vi "SVA 4MV5 PF CCSA RPJ SLJC.vi"() -> ()   [LabVIEW 2021]
uses:
  Control-Case.ctl
  <vilib>/vision/Image Controls.llb/IMAQ Image.ctl
  <vilib>/vision/NI_Vision_Development_Module.lvlib
panel:
  out "Aprobación de Lata":bool
  out "Distance 2":dbl[](graph) caption="Distancia entre perfil ideal y perfil real"
  out "Distance":dbl[](graph) caption="Distancia entre perfil ideal y perfil real"
  out "new picture 2":picture
  out "new picture":picture
  out "Datos finales":T1(array[cluster])
  in  "Crear patrón":bool
  in  "Concluir":bool
  in  "Lateral":bool
  in  "Superior":bool
  out "Fecha final":timestamp
  out "Rechazadas":dbl
  out "Aprobadas":dbl
  in  "Valor de aprobación Superiror":dbl=4.0 min=0.0 format="%.2f"
  out "Fecha inicio":timestamp
  out "Muestras":i32
  in  "Valor de aprobación Frontal":dbl=4.0 min=0.0 format="%.2f"
  # "Descripción:\nEste instrumento virtual permite detectar irregularidades en la geometría de latas de refresco usando el análisis de contornos:\n-Primeramente debe obtenerse un patrón para el perfil lateral e caso de no tenerlo, pues este se usará para detectar las irregularidades de capturas posteriores.\n-Como siguiente paso se toma una captura del perfil lateral y esta se desplegará en la imagen izquierda.\n-Como siguiente paso se toma una captura del perfil superior y esta se desplegará en la imagen derecha."
  # "Sistema de detección de defectos en latas \nbasado en el análisis de contornos\nProyecto de fin de semestre \nSistemas de visión artificial\nProfesor Erick Huitrón Ramírez"
  # "CUEVAS CERÓN SERGIO ALBERTO\nREYES PÉREZ JAVIER\nSALCEDO LICEA JUAN CARLOS"
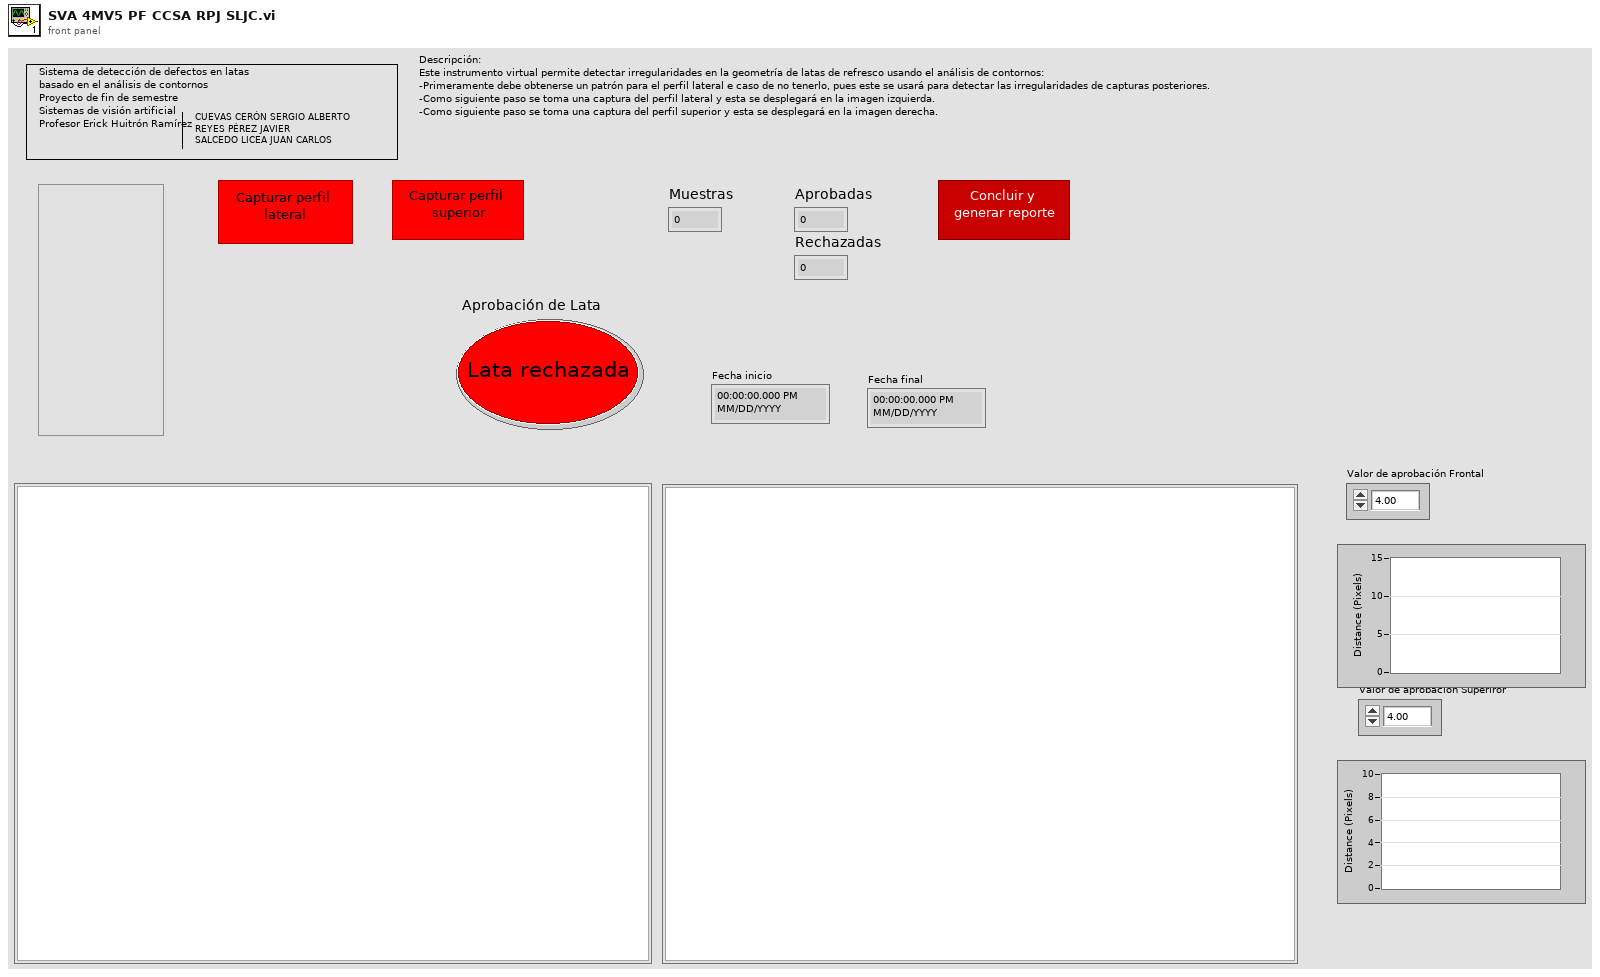
[diagram p1: front panel]
types:
  T1 = cluster{"Class":string, string, string, string}[]
  T2 = typedef "IMAQ Image.ctl" = refnum<image>
  T3 = typedef "Control-Case.ctl" = enum16{"Espera", "Patrón", "Toma lateral", "Toma superior", "Concluir"}
  T4 = enum16{"Rect Left To Right", "Rect Right To Left", "Rect Top To Bottom", "Rect Bottom To Top", "Annulus Inner To Outer", "Annulus Outer To Inner", "Annulus Start Angle To End Angle", "Annulus End Angle To Start Angle"}
  T5 = enum16{"Closest To Search Start", "Maximum Length", "Strongest Mean Gradient Change"}
  T6 = cluster{"Overlay?":bool, "Color":u32, "Width":u32, "Maintain Width?":bool}
  T7 = typedef "IMAQ Rectangle" = cluster{"Left":i32, "Top":i32, "Right":i32, "Bottom":i32, "Rotation":dbl}
  T8 = typedef "ROI Descriptor" = cluster{"Global Rectangle":i32[], "Contours":cluster{"ID":enum32{"External", "Internal"}, "Type":u32, "Coordinates":i32[]}[]}
  T9 = cluster{"Distance (Pixels)":dbl, "Distance (Real World)":dbl, "Angle (Absolute)":dbl, "Angle (Relative)":dbl}
  T10 = cluster{"Target Point":cluster{"X":dbl, "Y":dbl}, "Template Point":cluster{"X":dbl, "Y":dbl}, "Distance":dbl}[]
  T11 = cluster{"Center":cluster{"X":sgl, "Y":sgl}, "Radius":dbl, "Start Angle":dbl, "End Angle":dbl}
  T12 = cluster{"Class":string, "Distance (Pixels)":dbl, bool, dbl}
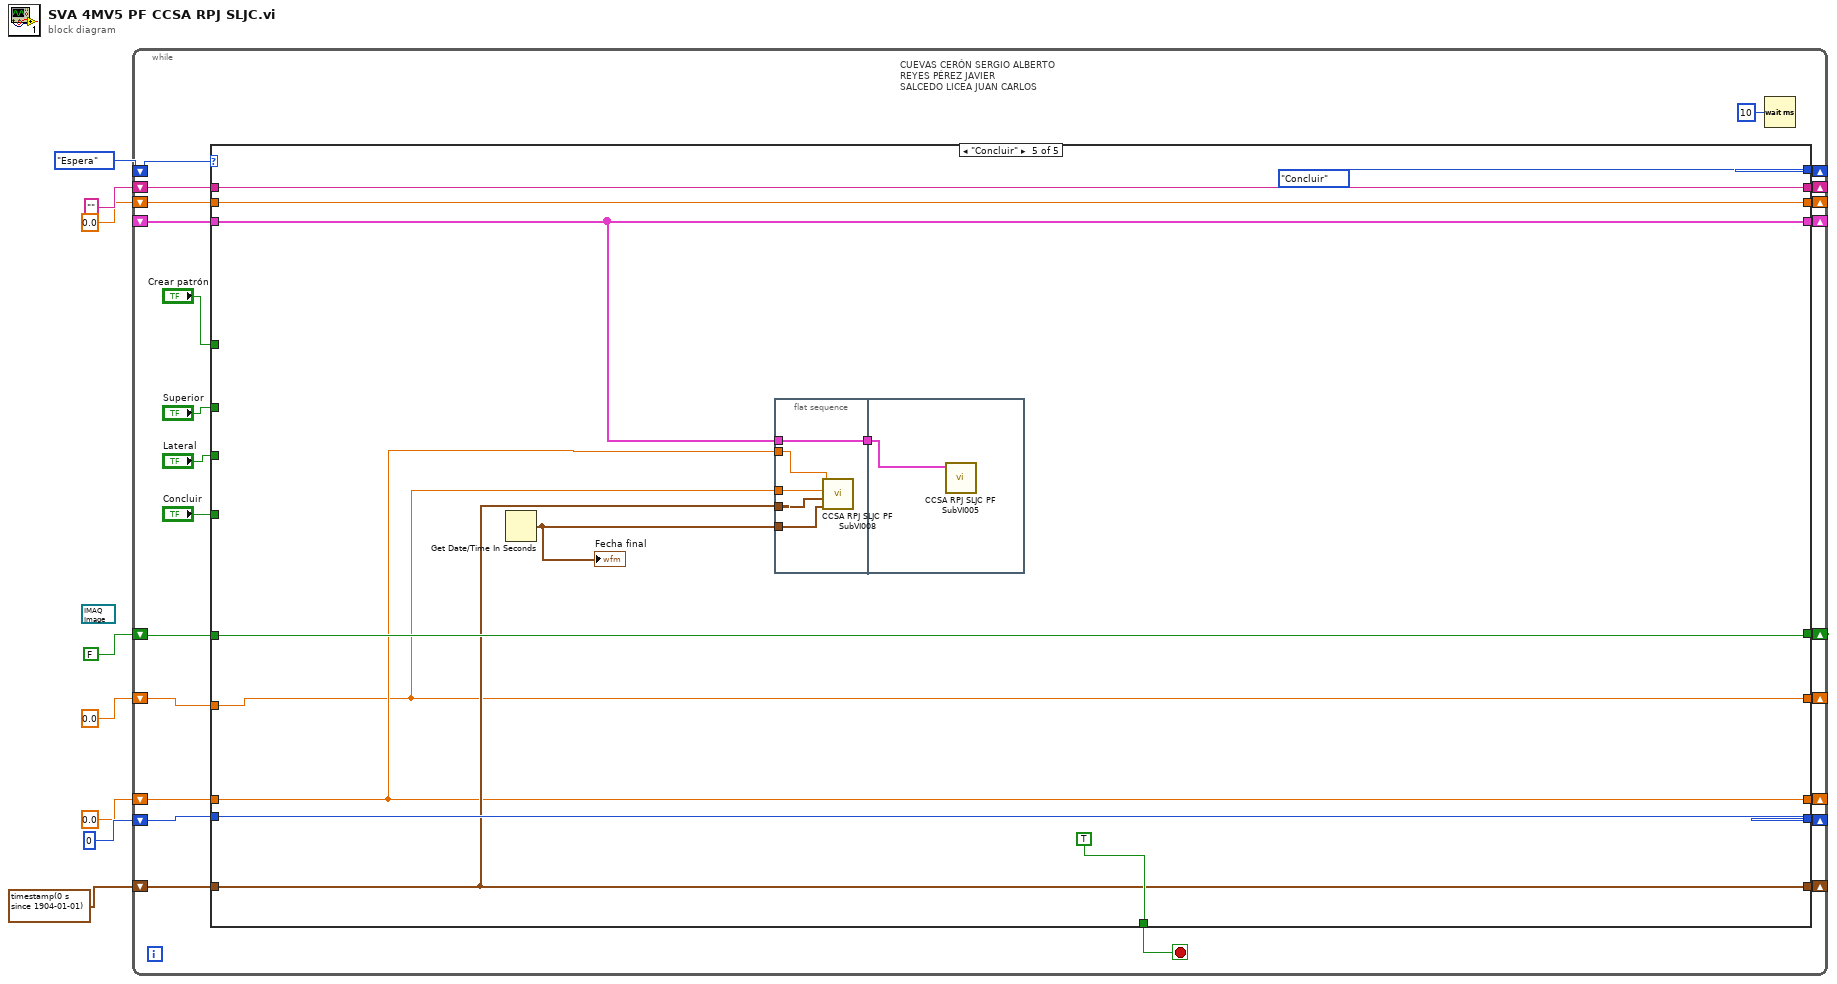
[diagram p0: block diagram]
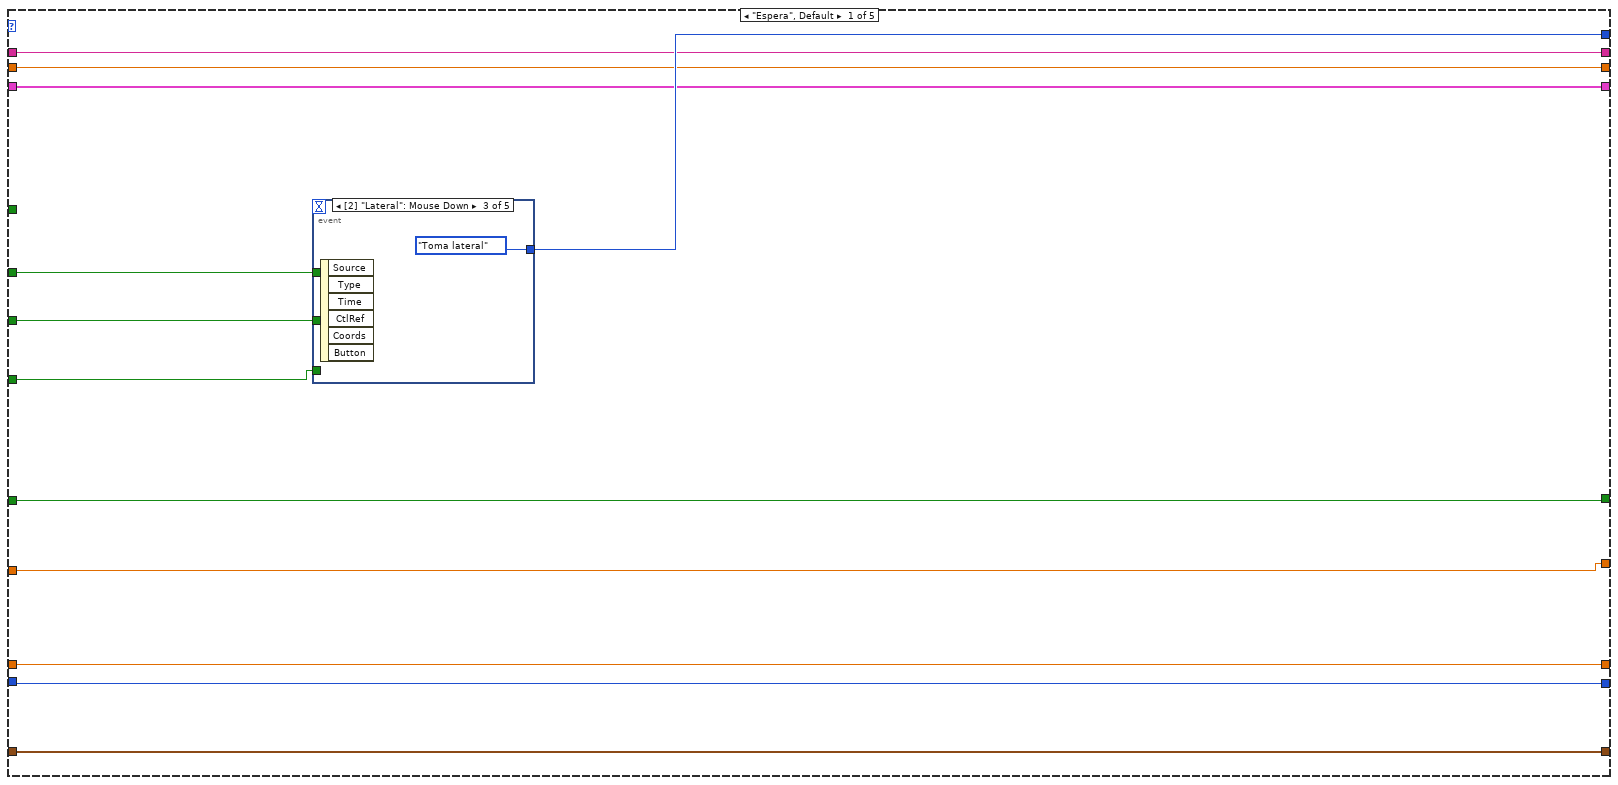
[diagram p2: hidden frame]
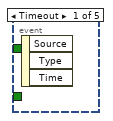
[diagram p3: hidden frame]
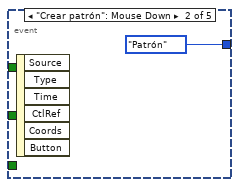
[diagram p4: hidden frame]
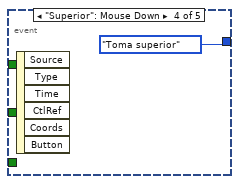
[diagram p5: hidden frame]
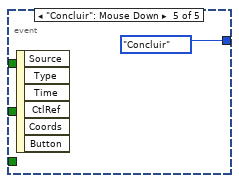
[diagram p6: hidden frame]
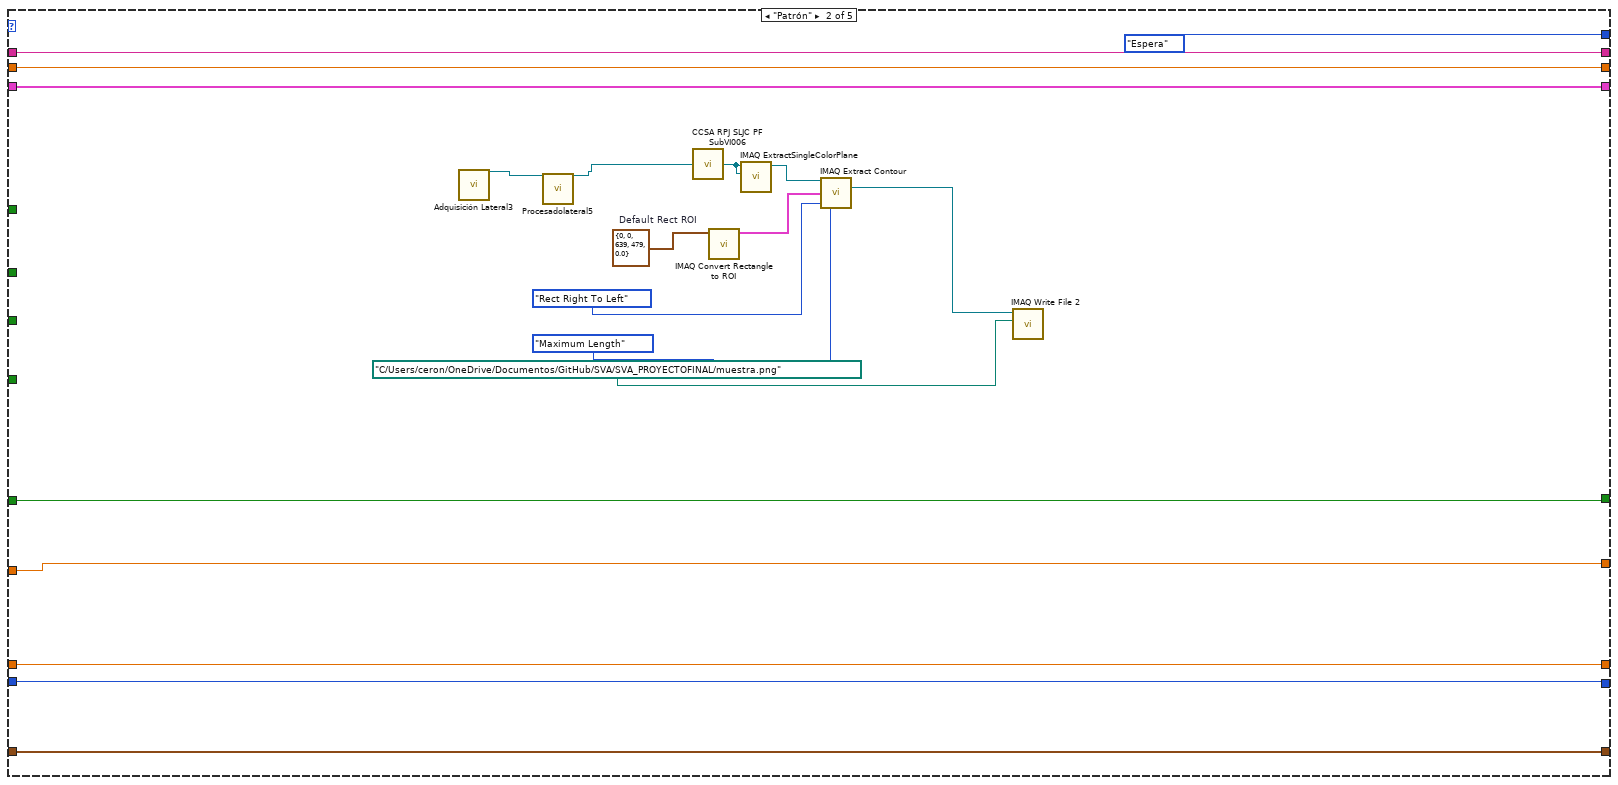
[diagram p7: hidden frame]
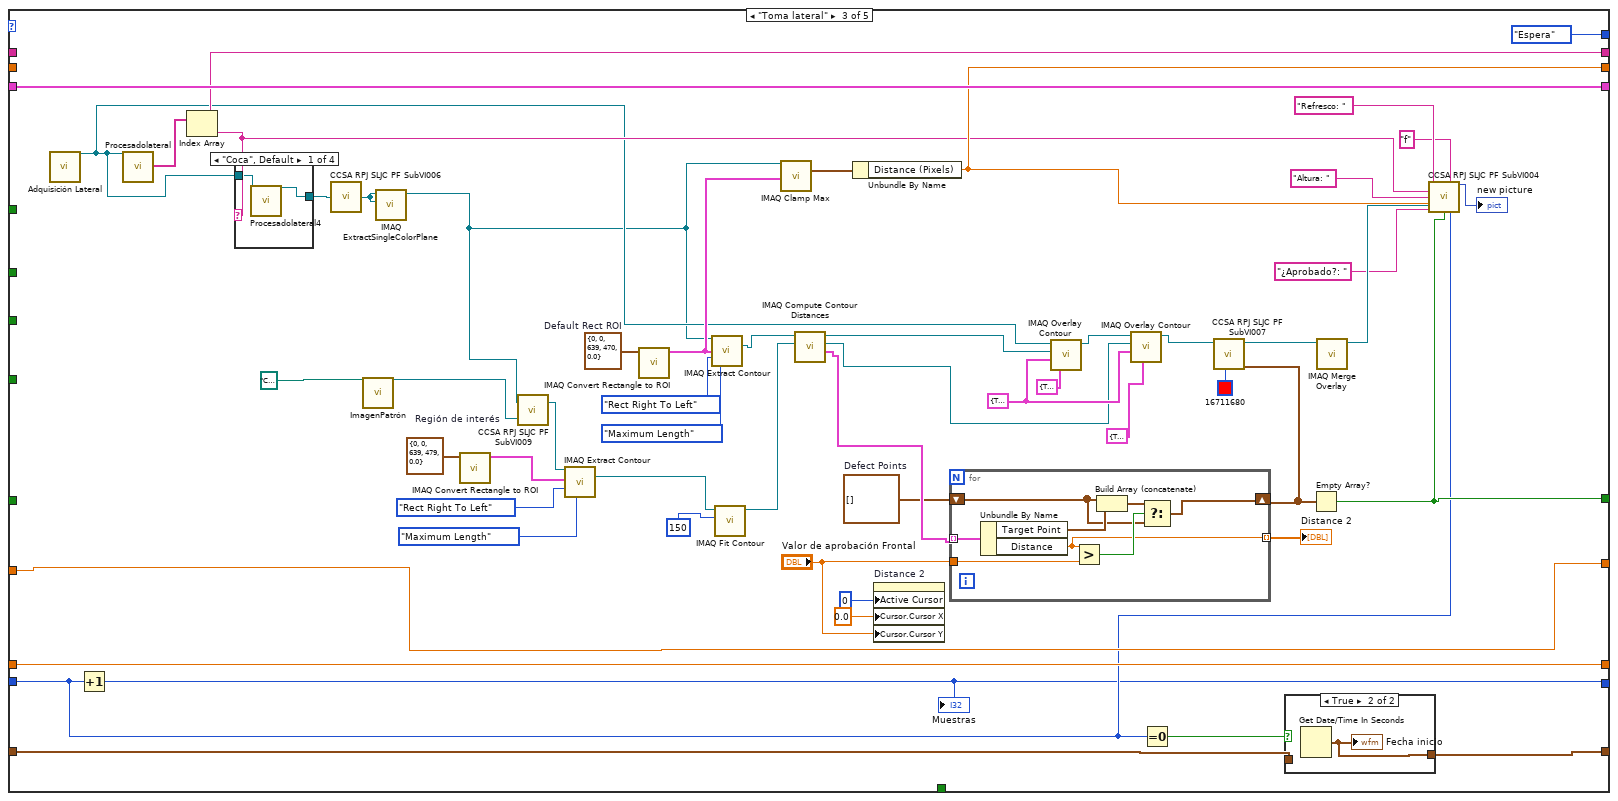
[diagram p8: hidden frame]
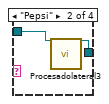
[diagram p10: hidden frame]
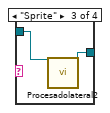
[diagram p11: hidden frame]
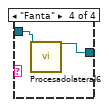
[diagram p12: hidden frame]
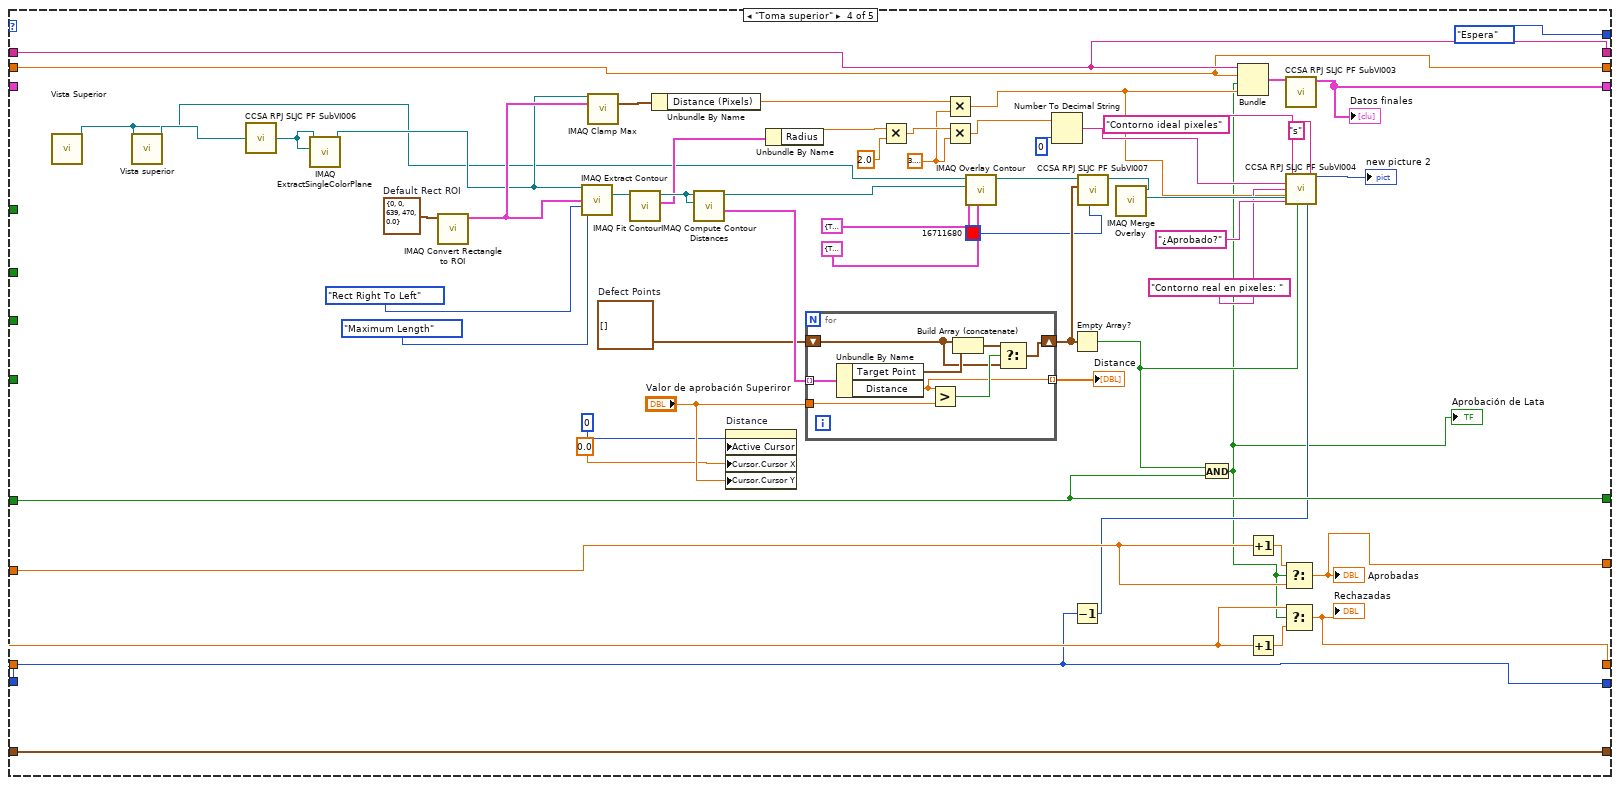
[diagram p13: hidden frame]
diagram:
  (unwired) T2 refnum ("Image Out (duplicate)")
  n1 = while {
    shift-right: [w32] -> _
    shift-left: Control-Case."Espera" -> [w31]
    shift-right: [w26] -> _
    shift-left: 0 ("x") -> [w25]
    shift-right: [w24] -> _
    shift-left: FALSE ("empty?") -> [w23]
    shift-right: [w22] -> _
    shift-left: 0.0 -> [w20]
    shift-right: [w21] -> _
    shift-left: 0.0 -> [w19]
    shift-right: [w17] -> _
    shift-left: 0.0 ("Distance (Pixels)") -> [w15]
    shift-right: [w18] -> _
    shift-left: "" ("Class") -> [w16]
    shift-right: [w14] -> _
    shift-left: _ -> [w13]
    shift-right: [w12] -> _
    shift-left: timestamp(0 s since 1904-01-01) ("seconds since 1Jan1904") -> [w11]
    stop <- w30 stop-if-true
    # "CUEVAS CERÓN SERGIO ALBERTO\nREYES PÉREZ JAVIER\nSALCEDO LICEA JUAN CARLOS"
    n2 = case shown="\"Concluir\"" w31 {
      tunnel: [w44 Control-Case."Espera" Control-Case."Espera" Control-Case."Espera" Control-Case."Concluir"] -> w32
      tunnel: [_ _ _ _ TRUE] -> w30
      tunnel: "Concluir" -> [w43 _ _ _ _]
      tunnel: "Lateral" -> [w42 _ _ _ _]
      tunnel: "Superior" -> [w41 _ _ _ _]
      tunnel: w25 -> [w37 w55 w75 w142 w214]
      tunnel: [w37 w55 w71 w142 w214] -> w26
      tunnel: [w40 w58 w82 w173 w213] -> w24
      tunnel: w23 -> [w40 w58 _ w173 w213]
      tunnel: [w39 w57 w93 w168 w206] -> w22
      tunnel: [w38 w56 w92 w167 w207] -> w21
      tunnel: w20 -> [w39 w57 w93 w175 w206]
      tunnel: w19 -> [w38 w56 w92 w174 w207]
      tunnel: [w36 w54 w84 w172 w212] -> w18
      tunnel: [w35 w53 w85 w171 w211] -> w17
      tunnel: w16 -> [w36 w54 _ w172 w212]
      tunnel: w15 -> [w35 w53 _ w171 w211]
      tunnel: [w34 w52 w86 w170 w209] -> w14
      tunnel: w13 -> [w34 w52 w86 _ w209]
      tunnel: [w33 w51 w91 w169 w208] -> w12
      tunnel: w11 -> [w33 w51 w90 w169 w208]
      tunnel: "Crear patrón" -> [_ _ _ _ _]
      frame "Espera", Default {
        n3 = event shown="[2] \"Lateral\": Mouse Down" {
          selector: _ -> [_ _ _ _ _]
          dyn-events: _ -> [_ _ _ _ _]
          timeout: _ -> [_ _ _ _ _]
          tunnel: w41 -> [_ _ _ _ _]
          tunnel: w42 -> [_ _ _ _ _]
          tunnel: w43 -> [_ _ _ _ _]
          tunnel: [_ Control-Case."Patrón" Control-Case."Toma lateral" Control-Case."Toma superior" Control-Case."Concluir"] -> w44
          event Timeout {
            n4 = event-data() -> ()  [unwired: 1 in, 3 out]
          }
          event "Crear patrón": Mouse Down {
            n5 = event-data() -> ()  [unwired: 1 in, 6 out]
          }
          event "Lateral": Mouse Down {
            n6 = event-data() -> ()  [unwired: 1 in, 6 out]
          }
          event "Superior": Mouse Down {
            n7 = event-data() -> ()  [unwired: 1 in, 6 out]
          }
          event "Concluir": Mouse Down {
            n8 = event-data() -> ()  [unwired: 1 in, 6 out]
          }
        }
      }
      frame "Patrón" {
        w64 = T7 {"Left"=0, "Top"=0, "Right"=639, "Bottom"=479, "Rotation"=0.0}  # Default Rect ROI
        n9 = call "Adquisición Lateral3"() -> ("Image Out"=w50:T2)  [unwired: 26 in, 1 out]
        n10 = call "Procesadolateral5"("Image In"=w50) -> ("Image Out"=w49:T2)  [unwired: 25 in, 1 out]
        n11 = call "CCSA RPJ SLJC PF SubVI006.vi"("Refnum in"=w49) -> ("Refnum out"=w60:T2)
        n12 = call "IMAQ Convert Rectangle to ROI"("Rectangle"=w64) -> ("ROI Descriptor"=w63:T8)  [unwired: 8 in, 1 out]
        n13 = call "IMAQ ExtractSingleColorPlane"("Image Dst"=w60, "Image Src"=w60) -> ("Image Dst Out"=w67:T2)  [unwired: 8 in, 1 out]
        n14 = call "IMAQ Extract Contour"("Source Image"=w67, "ROI Descriptor"=w63, "Search Direction"=T4."Rect Right To Left", "Contour Selection"=T5."Maximum Length") -> ("Contour Image Out"=w62:T2)  [unwired: 4 in, 7 out]
        n15 = call-poly "IMAQ Write File 2"("File Path"=path "C:/Users/ceron/OneDrive/Documentos/GitHub/SVA/SVA_PROYECTOFINAL/muestra.png" ("Imagen \nPatrón 2"), "Image"=w62) -> ()  [unwired: 8 in, 2 out]
      }
      frame "Toma lateral" {
        w95 = T7 {"Left"=0, "Top"=0, "Right"=639, "Bottom"=479, "Rotation"=0.0}  # Región de interés
        w96 = T7 {"Left"=0, "Top"=0, "Right"=639, "Bottom"=470, "Rotation"=0.0}  # Default Rect ROI
        w108 = cluster{"X":dbl, "Y":dbl}[] []  # Defect Points
        w104 = T6 {"Overlay?"=TRUE, "Color"=6618880, "Width"=3, "Maintain Width?"=TRUE} ("Contour Points Settings")
        n16 = call "Adquisición Lateral"() -> ("Image Out"=w70:T2)  [unwired: 26 in, 1 out]
        n17 = Increment(x=w75) -> (x+1=w71:i32)
        "Muestras" <- w71
        n18 = call "Procesadolateral"("Image In"=w70) -> ("Classes (TipoRefresco)"=w120:string[])  [unwired: 23 in, 3 out]
        n19 = Index Array(array=w120) -> (element=w84:string)  [unwired: 1 in]
        n20 = case shown="\"Coca\", Default" w84 {
          tunnel: w70 -> [w133 w136 w137 w139]
          tunnel: [w134 w135 w138 w140] -> w121
          frame "Coca", Default {
            n21 = call "Procesadolateral4"("Image In"=w133) -> ("Image Out"=w134:T2)  [unwired: 25 in, 1 out]
          }
          frame "Pepsi" {
            n22 = call "Procesadolateral3"("Image In"=w136) -> ("Image Out"=w135:T2)  [unwired: 25 in, 1 out]
          }
          frame "Sprite" {
            n23 = call "Procesadolateral2"("Image In"=w137) -> ("Image Out"=w138:T2)  [unwired: 25 in, 1 out]
          }
          frame "Fanta" {
            n24 = call "Procesadolateral6"("Image In"=w139) -> ("Image Out"=w140:T2)  [unwired: 25 in, 1 out]
          }
        }
        n25 = call "CCSA RPJ SLJC PF SubVI006.vi"("Refnum in"=w121) -> ("Refnum out"=w115:T2)
        n26 = call "ImagenPatrón"("Image Path"=path "C:/Users/ceron/OneDrive/Documentos/GitHub/SVA/SVA_PROYECTOFINAL/muestra.png" ("Imagen \nPatrón")) -> ("Image Out"=w73:T2)  [unwired: 25 in, 1 out]
        n27 = call "IMAQ ExtractSingleColorPlane"("Image Dst"=w115, "Image Src"=w115) -> ("Image Dst Out"=w69:T2)  [unwired: 8 in, 1 out]
        n28 = call "IMAQ Convert Rectangle to ROI"("Rectangle"=w95) -> ("ROI Descriptor"=w117:T8)  [unwired: 8 in, 1 out]
        n29 = call "CCSA RPJ SLJC PF SubVI009.vi"("Patrón original"=w73, "Toma original"=w69) -> ("Patrón corregido"=w72:T2)  [unwired: 1 out]
        n30 = call "IMAQ Extract Contour"("Source Image"=w72, "ROI Descriptor"=w117, "Search Direction"=T4."Rect Right To Left", "Contour Selection"=T5."Maximum Length") -> ("Contour Image Out"=w78:T2)  [unwired: 4 in, 7 out]
        n31 = call "IMAQ Convert Rectangle to ROI"("Rectangle"=w96) -> ("ROI Descriptor"=w118:T8)  [unwired: 8 in, 1 out]
        n32 = call "IMAQ Extract Contour"("Source Image"=w69, "ROI Descriptor"=w118, "Search Direction"=T4."Rect Right To Left", "Contour Selection"=T5."Maximum Length") -> ("Contour Image Out"=w110:T2)  [unwired: 4 in, 7 out]
        n33 = call-poly "IMAQ Fit Contour"("Control Points"=u32 150, "Contour Image"=w78) -> ("Contour Image Out"=w77:T2)  [unwired: 2 in, 7 out]
        n34 = call "IMAQ Clamp Max"("Source Image"=w69, "ROI Descriptor"=w118) -> ("Clamp Results"=w119:T9)  [unwired: 8 in, 5 out]
        n35 = call "IMAQ Compute Contour Distances"("Template Contour Image"=w77, "Target Contour Image"=w110) -> ("Distances"=w112:T10, "Template Contour Image Out (dup)"=w76:T2, "Target Contour Image Out (dup)"=w114:T2)  [unwired: 3 in, 4 out]
        n36 = Unbundle By Name(w119) -> ("Distance (Pixels)"=w85:dbl)
        n37 = property on="Distance 2" class="WFGraph (strict)"("Active Cursor"=u32 0, "Cursor.Cursor X"=0.0 ("Cursor.Cursor Position:Cursor X"), "Cursor.Cursor Y"="Valor de aprobación Frontal") -> ()  [unwired: 2 in, 2 out]
        n38 = for {
          tunnel: w112 -> [w125] mode=indexing
          shift-right: [w128] -> w116
          shift-left: w108 -> [w129]
          tunnel: [w127] -> w111 mode=indexing
          tunnel: "Valor de aprobación Frontal" -> [w126]
          n39 = Unbundle By Name(w125) -> ("Target Point"=w132:cluster{"X":dbl, "Y":dbl}, "Distance"=w127:dbl)
          n40 = Greater?(x=w127, y=w126) -> (0:w131:bool)
          n41 = Build Array (concatenate)(w129, w132) -> (w130:cluster{"X":dbl, "Y":dbl}[])
          n42 = Select(t=w130, s=w131, f=w129) -> (s? t:f=w128:cluster{"X":dbl, "Y":dbl}[])
        }
        "Distance 2" <- w111
        n43 = call "IMAQ Overlay Contour"("Contour Equation Settings"=T6 {"Overlay?"=TRUE, "Color"=3381759, "Width"=3, "Maintain Width?"=TRUE}, "Contour Points Settings"=w104, "Contour Image"=w114, "Image"=w70) -> ("Image Out"=w113:T2)  [unwired: 2 in, 5 out]
        n44 = call "IMAQ Overlay Contour"("Contour Equation Settings"=T6 {"Overlay?"=TRUE, "Color"=3381759, "Width"=3, "Maintain Width?"=TRUE}, "Contour Points Settings"=w104, "Contour Image"=w76, "Image"=w113) -> ("Image Out"=w89:T2)  [unwired: 2 in, 5 out]
        n45 = Equal To 0?(x=w75) -> (x = 0?=w122:bool)
        n46 = call "CCSA RPJ SLJC PF SubVI007.vi"("Color"=u32 16711680, "Points"=w116, "Image In"=w89) -> ("Image Out"=w88:T2)  [unwired: 7 in, 1 out]
        n47 = case shown="True" w122 {
          tunnel: [w123 w124] -> w91
          tunnel: w90 -> [w123 _]
          frame False {
          }
          frame True, Default {
            n48 = Get Date/Time In Seconds() -> (seconds since 1Jan1904=w124:timestamp)
            "Fecha inicio" <- w124
          }
        }
        n49 = Empty Array?(array=w116) -> (empty?=w82:bool)
        n50 = call "IMAQ Merge Overlay"("Image Src"=w88) -> ("Image Dst Out"=w87:T2)  [unwired: 9 in, 1 out]
        n51 = call "CCSA RPJ SLJC PF SubVI004.vi"("Dato"="Refresco: ", "Nombre imagen"="f", "Class"=w84, "Dato 2"="Altura: ", "Distance (Pixels)"=w85, "Dato 3"="¿Aprobado?: ", "Refnum in"=w87, "empty?"=w82, "number"=w75) -> ("new picture"=→"new picture":picture)  [unwired: 6 in]
      }
      frame "Toma superior" {
        w145 = 3.141592653589793
        w179 = T7 {"Left"=0, "Top"=0, "Right"=639, "Bottom"=470, "Rotation"=0.0}  # Default Rect ROI
        w187 = cluster{"X":dbl, "Y":dbl}[] []  # Defect Points
        n52 = call "Vista Superior"() -> ("Image Out"=w141:T2)  [unwired: 26 in, 1 out]
        n53 = call "Vista superior"("Image In"=w141) -> ("Image Out"=w197:T2)  [unwired: 25 in, 1 out]
        n54 = call "CCSA RPJ SLJC PF SubVI006.vi"("Refnum in"=w197) -> ("Refnum out"=w196:T2)
        n55 = call "IMAQ ExtractSingleColorPlane"("Image Dst"=w196, "Image Src"=w196) -> ("Image Dst Out"=w160:T2)  [unwired: 8 in, 1 out]
        n56 = call "IMAQ Convert Rectangle to ROI"("Rectangle"=w179) -> ("ROI Descriptor"=w165:T8)  [unwired: 8 in, 1 out]
        n57 = call "IMAQ Extract Contour"("Source Image"=w160, "ROI Descriptor"=w165, "Search Direction"=T4."Rect Right To Left", "Contour Selection"=T5."Maximum Length") -> ("Contour Image Out"=w189:T2)  [unwired: 4 in, 7 out]
        n58 = call "IMAQ Clamp Max"("Source Image"=w160, "ROI Descriptor"=w165) -> ("Clamp Results"=w166:T9)  [unwired: 8 in, 5 out]
        n59 = call-poly "IMAQ Fit Contour"("Contour Image"=w189) -> ("Circle"=w156:T11, "Contour Image Out"=w195:T2)  [unwired: 3 in, 6 out]
        n60 = Unbundle By Name(w166) -> ("Distance (Pixels)"=w146:dbl)
        n61 = call "IMAQ Compute Contour Distances"("Template Contour Image"=w195, "Target Contour Image"=w195) -> ("Distances"=w194:T10, "Target Contour Image Out (dup)"=w188:T2)  [unwired: 3 in, 5 out]
        n62 = property on="Distance" class="WFGraph (strict)"("Active Cursor"=u32 0, "Cursor.Cursor X"=0.0 ("Cursor.Cursor Position:Cursor X"), "Cursor.Cursor Y"="Valor de aprobación Superiror") -> ()  [unwired: 2 in, 2 out]
        n63 = Unbundle By Name(w156) -> ("Radius"=w150:dbl)
        n64 = for {
          tunnel: w194 -> [w205] mode=indexing
          shift-right: [w200] -> w191
          shift-left: w187 -> [w201]
          tunnel: [w199] -> w192 mode=indexing
          tunnel: "Valor de aprobación Superiror" -> [w198]
          n65 = Unbundle By Name(w205) -> ("Target Point"=w204:cluster{"X":dbl, "Y":dbl}, "Distance"=w199:dbl)
          n66 = Greater?(x=w199, y=w198) -> (0:w203:bool)
          n67 = Build Array (concatenate)(w201, w204) -> (w202:cluster{"X":dbl, "Y":dbl}[])
          n68 = Select(t=w202, s=w203, f=w201) -> (s? t:f=w200:cluster{"X":dbl, "Y":dbl}[])
        }
        "Distance" <- w192
        n69 = Multiply(x=w150, y=2.0) -> (x*y=w148:dbl)
        n70 = Multiply(x=w146, y=w145) -> (x*y=w144:dbl)
        n71 = Multiply(x=w148, y=w145) -> (x*y=w147:dbl)
        n72 = call "IMAQ Overlay Contour"("Contour Equation Settings"=T6 {"Overlay?"=TRUE, "Color"=3381759, "Width"=3, "Maintain Width?"=TRUE}, "Contour Points Settings"=T6 {"Overlay?"=TRUE, "Color"=6618880, "Width"=3, "Maintain Width?"=TRUE}, "Contour Image"=w188, "Image"=w141) -> ("Image Out"=w193:T2)  [unwired: 2 in, 5 out]
        n73 = Number To Decimal String(number=w147, width (-)=i16 0) -> (decimal integer string=w154:string)
        n74 = Empty Array?(array=w191) -> (empty?=w162:bool)
        n75 = Decrement(x=w142) -> (x-1=w158:i32)
        n76 = call "CCSA RPJ SLJC PF SubVI007.vi"("Color"=u32 16711680, "Points"=w191, "Image In"=w193) -> ("Image Out"=w163:T2)  [unwired: 7 in, 1 out]
        n77 = call "IMAQ Merge Overlay"("Image Src"=w163) -> ("Image Dst Out"=w159:T2)  [unwired: 9 in, 1 out]
        n78 = And(x=w162, y=w173) -> (x .and. y?=w143:bool)
        "Aprobación de Lata" <- w143
        n79 = Bundle("Class"=w172, "Distance (Pixels)"=w171, w143, w144) -> (w164:T12)  [unwired: 1 in]
        n80 = Increment(x=w175) -> (x+1=w177:dbl)
        n81 = Increment(x=w174) -> (x+1=w176:dbl)
        n82 = Select(t=w177, s=w143, f=w175) -> (s? t:f=w168:dbl)
        "Aprobadas" <- w168
        n83 = Select(t=w174, s=w143, f=w176) -> (s? t:f=w167:dbl)
        "Rechazadas" <- w167
        n84 = call "CCSA RPJ SLJC PF SubVI003.vi"("Datos"=w164) -> ("appended array"=w170:T1)  [unwired: 10 in]
        "Datos finales" <- w170
        n85 = call "CCSA RPJ SLJC PF SubVI004.vi"("Dato"="Contorno ideal pixeles", "Nombre imagen"="s" ("string"), "Class"=w154, "Dato 2"="Contorno real en pixeles: ", "Distance (Pixels)"=w144, "Dato 3"="¿Aprobado?", "Refnum in"=w159, "empty?"=w162, "number"=w158) -> ("new picture"=→"new picture 2":picture)  [unwired: 6 in]
      }
      frame "Concluir" {
        n86 = Get Date/Time In Seconds() -> (seconds since 1Jan1904=w217:timestamp)
        "Fecha final" <- w217
        n87 = flat-sequence {
          tunnel: w217 -> [w222]
          tunnel: w209 -> [w221]
          tunnel: [w221] -> w210
          tunnel: w208 -> [w220]
          tunnel: w207 -> [w219]
          tunnel: w206 -> [w218]
          tunnel: w210 -> [w223]
          frame #0 {
            n88 = call "CCSA RPJ SLJC PF SubVI008.vi"("Final"=w222, "Inicio"=w220, "Numeric"=w218, "Numeric 2"=w219) -> ()  [unwired: 8 in]
          }
          frame #1 {
            n89 = call "CCSA RPJ SLJC PF SubVI005.vi"("Datos finales"=w223) -> ()  [unwired: 11 in]
          }
        }
      }
    }
    n90 = Wait (ms)(milliseconds to wait=u32 10) -> ()  [unwired: 1 out]
  }
